vi "niRFSysCalReader Interpolation Enabled.vi"(8 "error in":errorcluster, 10 "Enable Interpolation?":bool=TRUE, 11 "niRFSysCalReader Handle":T1) -> (0 "error out":errorcluster, 3 "niRFSysCalReader Handle out":T1)   [LabVIEW 2016, in "niRFSysCalReader.lvlib"]
doc: "Specifies if an interpolation should be performed, when fetching the offsets for uncalibrated settings."
uses:
  niRFSysCalReader.lvlib
  _INCLUDES/niRFSysCalReader Handle.ctl
  _INCLUDES/niRFSysCalReader Core States.ctl
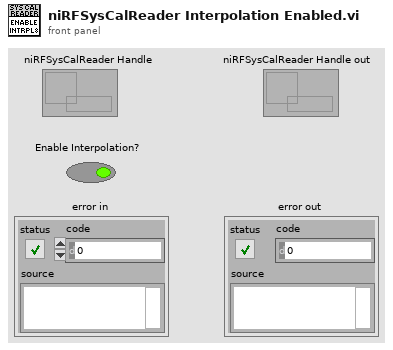
[diagram p1: front panel]
types:
  T1 = typedef "niRFSysCalReader.lvlib/niRFSysCalReader Handle.ctl" = refnum<data-value>
  T2 = typedef "niRFSysCalReader.lvlib/niRFSysCalReader Core States.ctl" = enum16{"Initialize", "Interpolator State", "Add Pathloss", "Get Pathloss", "Remove Pathloss", "Close"}
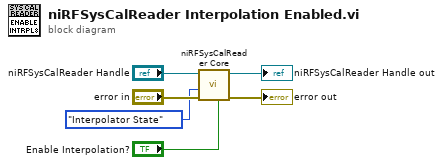
[diagram p0: block diagram]
diagram:
  n1 = call "niRFSysCalReader Core.vi"("Enable Interpolation?"="Enable Interpolation?", "error in"="error in", "niRFSysCalReader State"=niRFSysCalReader_Core_States."Interpolator State", "niRFSysCalReader Handle"="niRFSysCalReader Handle") -> ("error out"=→"error out":errorcluster, "niRFSysCalReader Handle out"=→"niRFSysCalReader Handle out":T1)  [unwired: 5 in, 1 out]
